vi "Change the Port Number for TCP to Dashboard.vi"(10 "Update":bool) -> (2 "Port Number":i64)   [LabVIEW 2023]
uses:
  <vilib>/Rock Robotics/Network Tables/NT Write Integer.vi
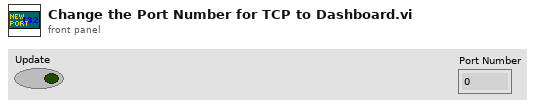
[diagram p1: front panel]
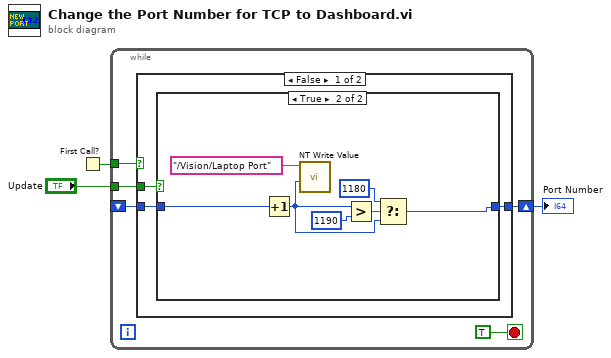
[diagram p0: block diagram]
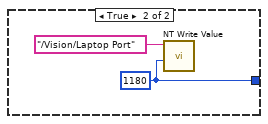
[diagram p3: hidden frame]
diagram:
  n1 = First Call?() -> (First Call?: T/F=w1:bool)
  n2 = while {
    tunnel: "Update" -> [w7]
    shift-right: [w5] -> w2
    shift-left: _ -> [w6]
    tunnel: w1 -> [w4]
    stop <- TRUE stop-if-true
    n3 = case shown="False" w4 {
      tunnel: w7 -> [w11 _]
      tunnel: w6 -> [w10 _]
      tunnel: [w9 w20] -> w5
      frame False {
        n4 = case shown="True" w11 {
          tunnel: w10 -> [w12 w18]
          tunnel: [w12 w13] -> w9
          frame False {
          }
          frame True {
            n5 = Increment(x=w18) -> (x+1=w15:i64)
            n6 = call-poly <vilib>:"NT Write Value.vi"("value"=w15, "name"="/Vision/Laptop Port" ("Name")) -> ()  [unwired: 9 in, 1 out]
            n7 = Greater?(x=w15, y=i64 1190) -> (0:w16:bool)
            n8 = Select(t=i64 1180, s=w16, f=w15) -> (s? t:f=w13:i64)
          }
        }
      }
      frame True {
        w20 = i64 1180
        n9 = call-poly <vilib>:"NT Write Value.vi"("value"=w20, "name"="/Vision/Laptop Port" ("Name")) -> ()  [unwired: 9 in, 1 out]
      }
    }
  }
  "Port Number" <- w2
